vi "Falcon_astrom_test.vi"() -> ()   [LabVIEW 2011]
panel:
  in  "Inversion Cluster":T1={"Invert Angle"=FALSE, "Invert X"=TRUE, "Invert Y"=TRUE}
  out "Corresponding Y":dbl
  out "Corresponding X":dbl
  in  "Requested DEC":dbl format="%<%H:%M:%S>t"
  in  "Requested RA":dbl format="%<%H:%M:%S%1u>t"
  out "Pixel DEC":dbl format="%<%H:%M:%S%2u>t"
  out "Pixel RA":dbl format="%<%H:%M:%S%3u>t"
  in  "DECsonde":dbl format="%<%H:%M:%S>t"
  in  "RAsonde":dbl format="%<%H:%M:%S%1u>t"
  in  "Pixel Y":dbl
  in  "Pixel X":dbl
  in  "Rotation":dbl format="%.1f"
  in  "Binning":u16(ring)=2 items=["1 x 1"=1, "2 x 2"=2, "4 x 4"=4, "5 x 5"=5]
  in  "PIXSCALE":cluster{"pixscale2":dbl, "pixscale1":dbl}={"pixscale2"=0.1288, "pixscale1"=0.1288}
  in  "NAXIS":cluster{"naxis2":u16, "naxis1":u16}={"naxis2"=1000, "naxis1"=1000}
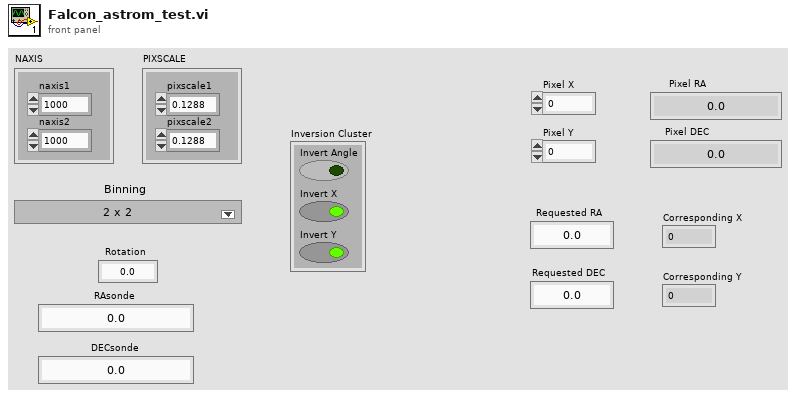
[diagram p1: front panel]
types:
  T1 = cluster{"Invert Angle":bool, "Invert X":bool, "Invert Y":bool}
  T2 = cluster{"NAXIS":dbl[], "CD":dbl[][], "CDELT":dbl[], "CRPIX":dbl[], "CTYPE":string[], "CRVAL":dbl[], "LONGPOLE":dbl, "LATPOLE":dbl, "PV2":dbl[]}
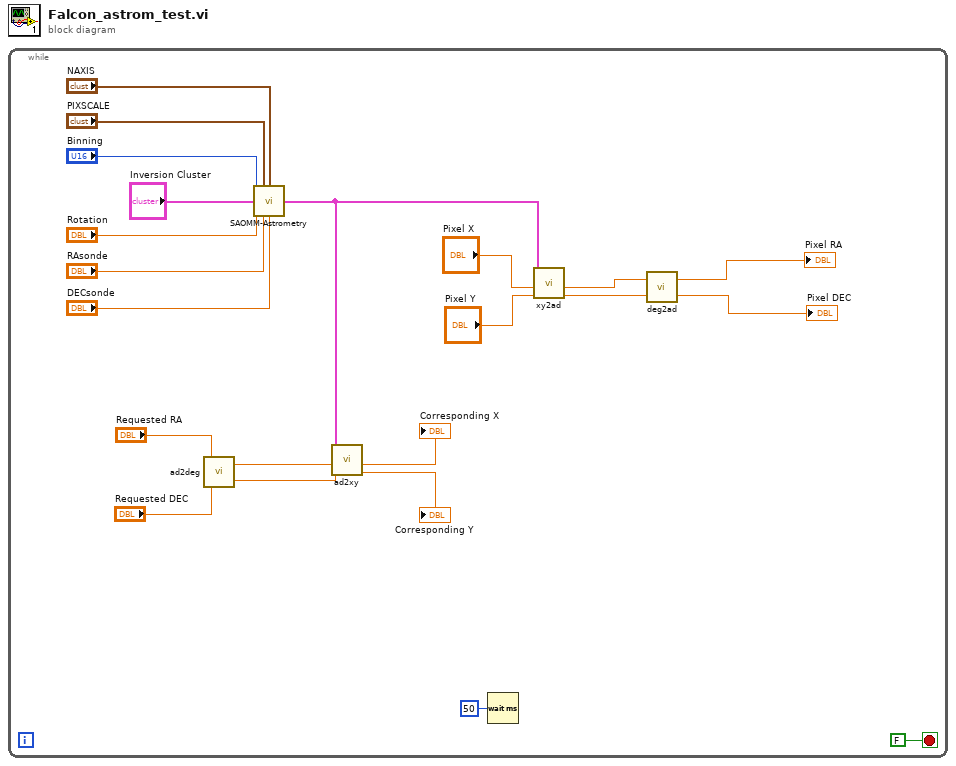
[diagram p0: block diagram]
diagram:
  n1 = while {
    stop <- FALSE stop-if-true
    n2 = call "ad2deg.vi"("DEC (sec)"="Requested DEC", "RA (sec)"="Requested RA") -> ("DEC (°)"=w10:dbl, "RA (°)"=w11:dbl)
    n3 = call "SAOMM-Astrometry.vi"("Binning"="Binning", "PIXSCALE"="PIXSCALE", "NAXIS"="NAXIS", "Inversion Cluster"="Inversion Cluster", "Rotation"="Rotation", "RAsonde"="RAsonde", "DECsonde"="DECsonde") -> ("GuideAstrom"=w7:T2)  [unwired: 8 in]
    n4 = call "ad2xy.vi"("DEC"=w10, "RA"=w11, "Astrometry"=w7) -> ("Y"=→"Corresponding Y":dbl, "X"=→"Corresponding X":dbl)  [unwired: 6 in, 1 out]
    n5 = Wait (ms)(milliseconds to wait=u32 50) -> ()  [unwired: 1 out]
    n6 = call "xy2ad.vi"("Y (px)"="Pixel Y", "X (px)"="Pixel X", "Astrometry"=w7) -> ("DEC (°)"=w3:dbl, "RA (°)"=w4:dbl)  [unwired: 5 in, 2 out]
    n7 = call "deg2ad.vi"("DEC (°)"=w3, "RA (°)"=w4) -> ("DEC (°)"=→"Pixel DEC":dbl, "RA (sec)"=→"Pixel RA":dbl)
  }
